vi "DefendGoalTactic.vi"(7 "First call?":bool=TRUE, 8 "error in (no error)":errorcluster, 9 "Robot":refnum<class "Robot.lvclass">, 10 "Game":refnum<class "Game.lvclass">, 11 "DefendGoalTactic in":refnum<class "DefendGoalTactic.lvclass">) -> (0 "error out":errorcluster, 2 "Robot out":refnum<class "Robot.lvclass">, 3 "DefendGoalTactic out":refnum<class "DefendGoalTactic.lvclass">)   [LabVIEW 2023, in "DefendGoalTactic.lvclass"]
uses:
  DefendGoalTactic.lvclass
  Robot_class/Robot.lvclass
  Game_class/Game.lvclass
  Robot_class/tactics.ctl
  Tactic_class/Tactic.lvclass/Tactic.ctl
  Skillbook_class/Skillbook.lvclass/Skillbook.ctl
  Game_class/Game.lvclass/Game.ctl
  Parameters_class/Parameters.lvclass/Parameters.ctl
  Robot_class/Robot.lvclass/Robot.ctl
  Game_class/Read FieldRef.vi
  Game_class/Read Utilities.lvclass.vi
  Game_class/Read Parameters.lvclass.vi
  Parameters_class/Read AttakingOurselves.vi
  Skillbook_class/Read KickToSkill.vi
  Tactic_class/Read Skillbook.vi
  Robot_class/Write tactic.vi
  Skillbook_class/Skillbook.lvclass
  DefBallTrajSkill_class/DefBallTrajSkill.lvclass
  DefBallEnemySkill_class/DefBallEnemySkill.lvclass
  DefBallOrientSkill_class/DefBallOrientSkill.lvclass
  Field_class/Field.lvclass
  Utilities_class/Utilities.lvclass
  Parameters_class/Parameters.lvclass
  KickToSkill_class/KickToSkill.lvclass
panel:
  out "x .or. y?":bool
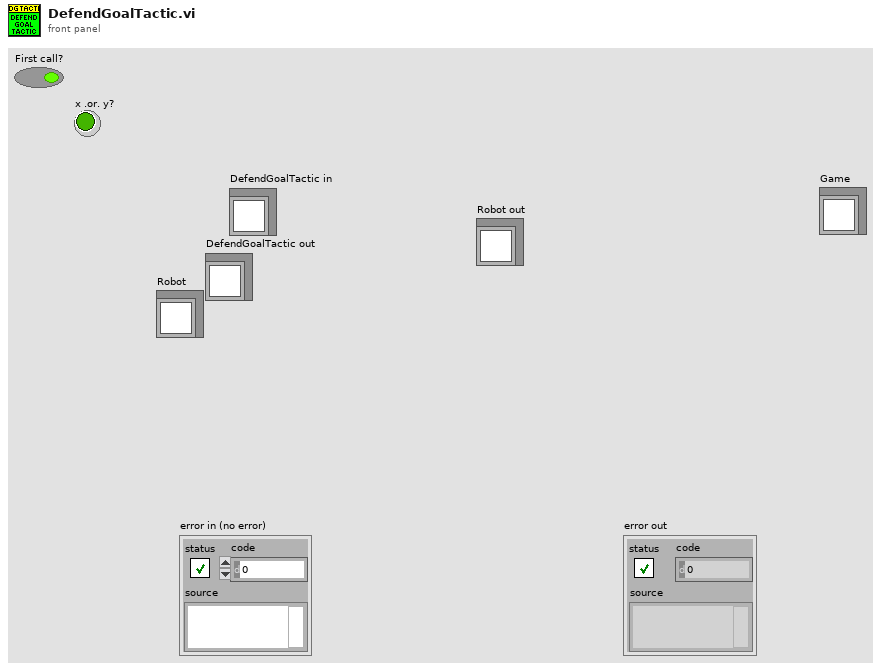
[diagram p1: front panel]
types:
  T1 = enum16{"State 0", "State 1", "State 2", "State 3", "Exit"}
  T2 = typedef "tactics.ctl" = enum16{"ReceivePassInFuturePoint", "Roller", "PrepareRollToPassRollerGoTo", "PrepareRollToPassReceiverGoTo", "WaitRoll", "PositionToRoll", "PenaltyAttacker", "PassObserver", "PenaltyDefense", "TableReceiverTactic", "Test", "DefendGoal", "Marker", "FollowAttacker", "DefendArea", "Shoot", "AttackerAimGoal", "AttackerBallOutOfField", "AttackerBlock", "AttackerStop", "Duelist", "Halt", "ZigZag", "GoTo", "Timeout", "KickToPassReceiver", "PositionToReceivePass", "DefendAreaVSS", "DefendGoalVSS", "KickVSS", "AttackVSS", "DispBallVSS", "PenaltyAttackVSS", "WaitPass"}
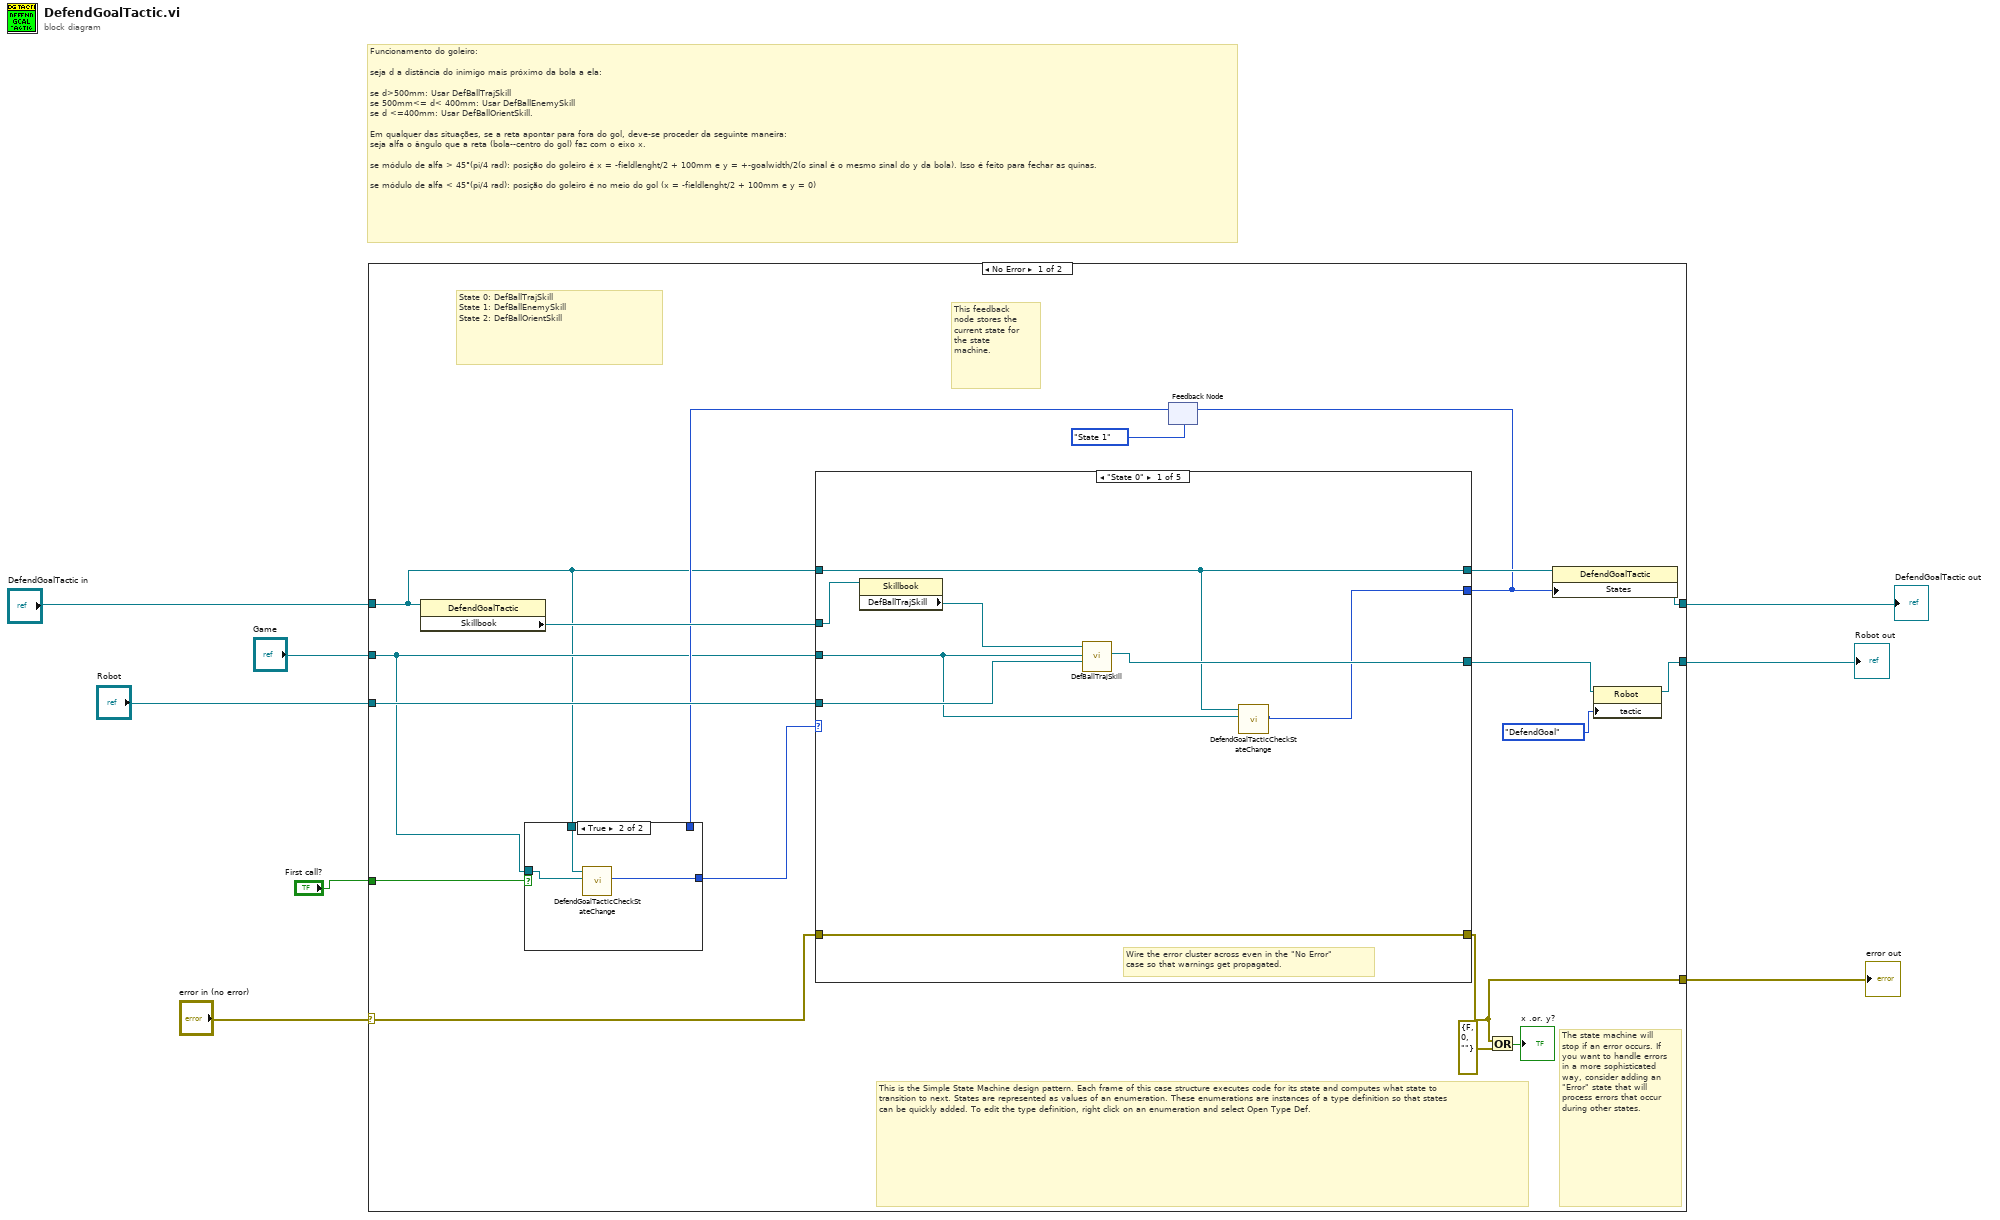
[diagram p0: block diagram]
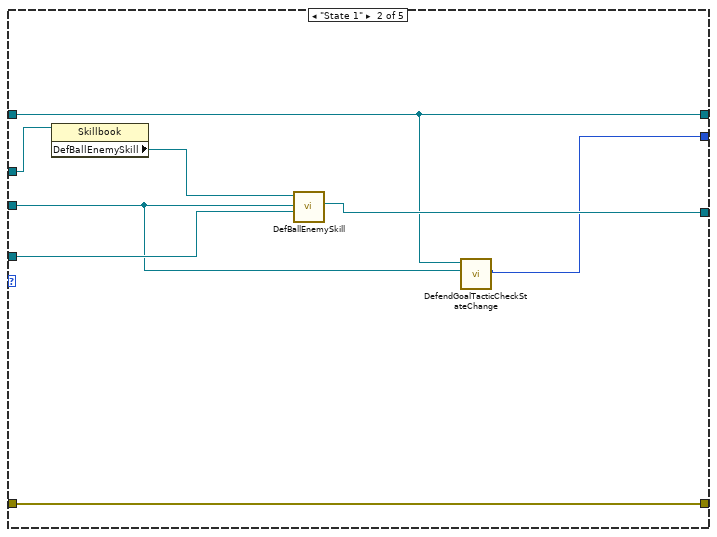
[diagram p3: hidden frame]
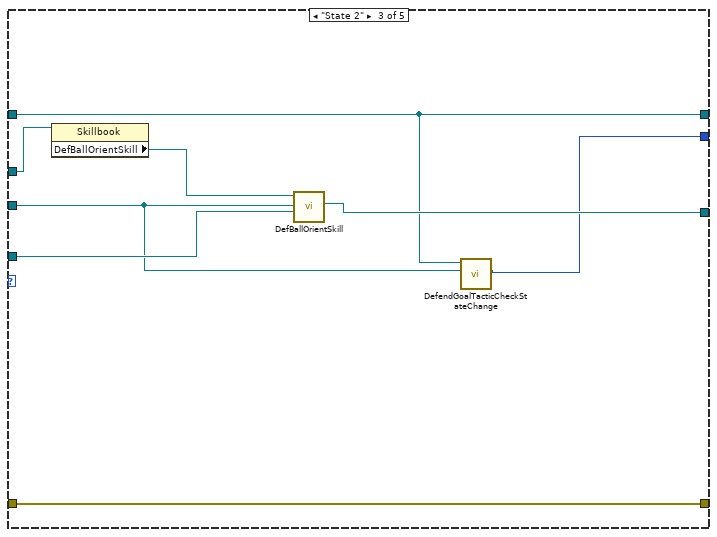
[diagram p4: hidden frame]
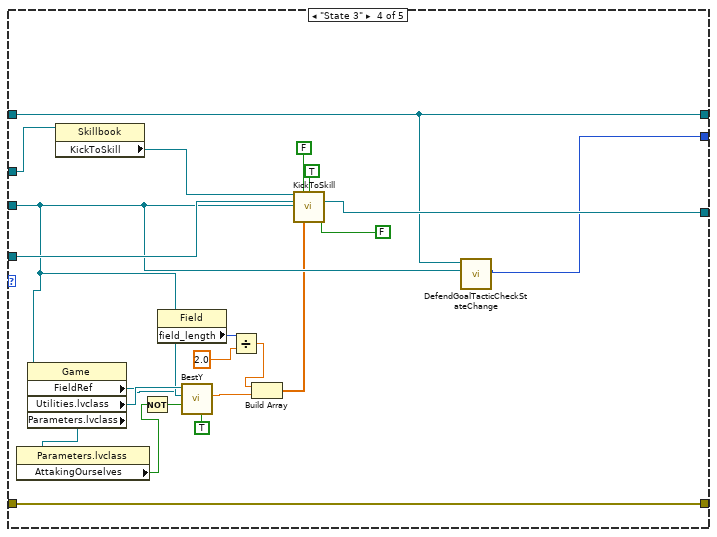
[diagram p5: hidden frame]
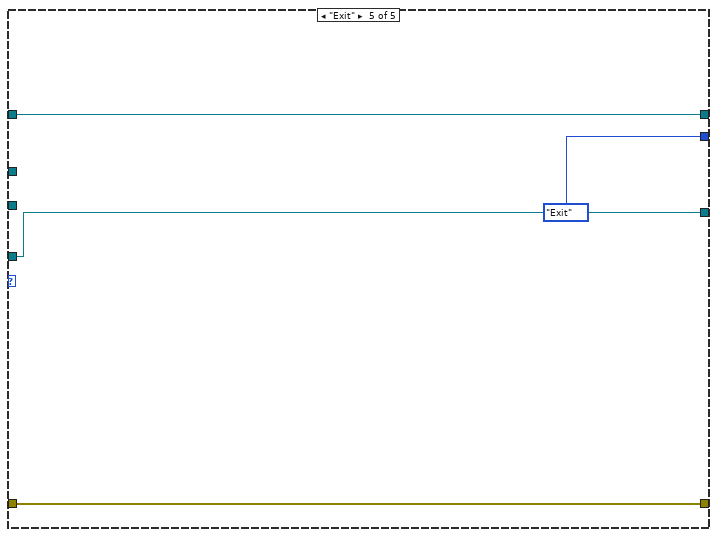
[diagram p6: hidden frame]
diagram:
  # "Funcionamento do goleiro:\n\nseja d a distância do inimigo mais próximo da bola a ela:\n\nse d>500mm: Usar DefBallTrajSkill\nse 500mm<= d< 400mm: Usar DefBallEnemySkill\nse d <=400mm: Usar DefBallOrientSkill.\n\nEm qualquer das situações, se a reta apontar para fora do gol, deve-se proceder da seguinte maneira:\nseja alfa o ângulo que a reta (bola--centro do gol) faz com o eixo x.\n\nse módulo de alfa > 45°(pi/4 rad): posição do goleiro é x = -fieldlenght/2 + 100mm e y = +-goalwidth/2(o sinal é o mesmo sinal do y da bola). Isso é feito para fechar as quinas.\n\nse módulo de alfa < 45°(pi/4 rad): posição do goleiro é no meio do gol (x = -fieldlenght/2 + 100mm e y = 0)"
  n1 = case shown="No Error" "error in (no error)" {
    selector: "error in (no error)" -> [w25 w83]
    tunnel: [w24 w83] -> w7
    tunnel: [w20 w82] -> w2
    tunnel: "DefendGoalTactic in" -> [w16 w82]
    tunnel: "Robot" -> [w23 w81]
    tunnel: [w13 w81] -> w5
    tunnel: "Game" -> [w18 _]
    tunnel: "First call?" -> [w10 _]
    frame No Error {
      # "State 0: DefBallTrajSkill\nState 1: DefBallEnemySkill\nState 2: DefBallOrientSkill"
      # "The state machine will stop if an error occurs. If you want to handle errors in a more sophisticated way, consider adding an \"Error\" state that will process errors that occur during other states."
      # "This feedback node stores the current state for the state machine."
      # "This is the Simple State Machine design pattern. Each frame of this case structure executes code for its state and computes what state to transition to next. States are represented as values of an enumeration. These enumerations are instances of a type definition so that states can be quickly added. To edit the type definition, right click on an enumeration and select Open Type Def."
      # "Wire the error cluster across even in the \"No Error\"\ncase so that warnings get propagated."
      n2 = property class="DefendGoalTactic"(reference=w16) -> ("Skillbook"=w22:refnum<class "Skillbook.lvclass">)  [unwired: 1 in, 2 out]
      n3 = feedback #1(T1."State 1" ("States")) -> (w19:T1)
      n4 = case shown="True" w10 {
        tunnel: [w27 w30] -> w9
        tunnel: w19 -> [w27 _]
        tunnel: w18 -> [_ w29]
        tunnel: w16 -> [_ w28]
        frame False {
        }
        frame True {
          n5 = call "DefendGoalTacticCheckStateChange.vi"("Game"=w29, "DefendGoalTactic in"=w28) -> ("States"=w30:T1)  [unwired: 7 in, 2 out]
        }
      }
      n6 = case shown="\"State 0\"" w9 {
        tunnel: w25 -> [w38 w46 w54 w76 w80]
        tunnel: [w38 w46 w54 w76 w80] -> w24
        tunnel: w22 -> [w34 w42 w50 w72 _]
        tunnel: w23 -> [w36 w44 w52 w74 w77]
        tunnel: [w35 w43 w51 w73 w77] -> w14
        tunnel: [w31 w39 w47 w70 w79] -> w21
        tunnel: w16 -> [w31 w39 w47 w70 w79]
        tunnel: w18 -> [w32 w40 w48 w65 _]
        tunnel: [w33 w41 w49 w71 T1."Exit" ("States")] -> w12
        frame "State 0" {
          n7 = property class="Skillbook"(reference=w34) -> ("DefBallTrajSkill"=w37:refnum<class "DefBallTrajSkill.lvclass">)  [unwired: 1 in, 2 out]
          n8 = call "DefBallTrajSkill.vi"("Robot"=w36, "Game"=w32, "DefBallTrajSkill in"=w37) -> ("robot out"=w35:refnum<class "Robot.lvclass">)  [unwired: 6 in, 2 out]
          n9 = call "DefendGoalTacticCheckStateChange.vi"("Game"=w32, "DefendGoalTactic in"=w31) -> ("States"=w33:T1)  [unwired: 7 in, 2 out]
        }
        frame "State 1" {
          n10 = property class="Skillbook"(reference=w42) -> ("DefBallEnemySkill"=w45:refnum<class "DefBallEnemySkill.lvclass">)  [unwired: 1 in, 2 out]
          n11 = call "DefBallEnemySkill.vi"("Robot"=w44, "Game"=w40, "DefBallEnemySkill in"=w45) -> ("robot out"=w43:refnum<class "Robot.lvclass">)  [unwired: 6 in, 2 out]
          n12 = call "DefendGoalTacticCheckStateChange.vi"("Game"=w40, "DefendGoalTactic in"=w39) -> ("States"=w41:T1)  [unwired: 7 in, 2 out]
        }
        frame "State 2" {
          n13 = property class="Skillbook"(reference=w50) -> ("DefBallOrientSkill"=w53:refnum<class "DefBallOrientSkill.lvclass">)  [unwired: 1 in, 2 out]
          n14 = call "DefBallOrientSkill.vi"("Robot"=w52, "Game"=w48, "DefBallOrientSkill in"=w53) -> ("Robot out"=w51:refnum<class "Robot.lvclass">)  [unwired: 6 in, 2 out]
          n15 = call "DefendGoalTacticCheckStateChange.vi"("Game"=w48, "DefendGoalTactic in"=w47) -> ("States"=w49:T1)  [unwired: 7 in, 2 out]
        }
        frame "State 3" {
          n16 = property class="Game"(reference=w65) -> ("FieldRef"=w59:refnum<class "Field.lvclass">, "Utilities.lvclass"=w66:refnum<class "Utilities.lvclass">, "Parameters.lvclass"=w64:refnum<class "Parameters.lvclass">)  [unwired: 1 in, 2 out]
          n17 = property class="Parameters.lvclass"(reference=w64) -> ("AttakingOurselves"=w62:bool)  [unwired: 1 in, 2 out]
          n18 = property class="Skillbook"(reference=w72) -> ("KickToSkill"=w75:refnum<class "KickToSkill.lvclass">)  [unwired: 1 in, 2 out]
          n19 = Not(x=w62) -> (.not. x?=w63:bool)
          n20 = property class="Field"(reference=w59) -> ("field_length"=w58:i32)  [unwired: 1 in, 2 out]
          n21 = call "BestY.vi"("Utilities in"=w66, "Game"=w65, "inimigos"=w63, "Goalie?"=TRUE) -> ("Best y"=w61:dbl)  [unwired: 1 in, 4 out]
          n22 = Divide(x=w58, y=2.0) -> (x/y=w56:dbl)
          n23 = Build Array(w56, w61) -> (w60:dbl[])
          n24 = call "KickToSkill.vi"("KickToSkill in"=w75, "use criteria?"=FALSE, "chipKick ?"=TRUE, "Robot"=w74, "Game"=w65, "calculate force?"=FALSE, "Target"=w60) -> ("Robot out"=w73:refnum<class "Robot.lvclass">)  [unwired: 6 in, 2 out]
          n25 = call "DefendGoalTacticCheckStateChange.vi"("Game"=w65, "DefendGoalTactic in"=w70) -> ("States"=w71:T1)  [unwired: 7 in, 2 out]
        }
        frame "Exit" {
        }
      }
      n26 = feedback-in #1(w12) -> ()
      n27 = Or(x=w24, y=errorcluster {"status"=FALSE, "code"=0, "source"=""}) -> (x .or. y?=→"x .or. y?":bool)
      n28 = property class="DefendGoalTactic"(reference=w21, "States"=w12) -> (reference out=w20:refnum<class "DefendGoalTactic.lvclass">)  [unwired: 1 in, 1 out]
      n29 = property class="Robot"(reference=w14, "tactic"=tactics."DefendGoal") -> (reference out=w13:refnum<class "Robot.lvclass">)  [unwired: 1 in, 1 out]
    }
    frame Error {
    }
  }
  "error out" <- w7
  "Robot out" <- w5
  "DefendGoalTactic out" <- w2
